vi "Create LVObjectMsg.vi"(8 "error in (no error)":errorcluster, 10 "Message Data":refnum<class>, 11 "Message Name":string) -> (0 "error out":errorcluster, 3 "LVObjectMsg out":refnum<class "LVObjectMsg.lvclass">)   [LabVIEW 2018, in "LapDog.Messaging.v3.NativeTypes.lvlib" / "LVObjectMsg.lvclass"]
doc: "Returns a LVObjectMsg object with the given name.\n\nThis method executes regardless of the error in state."
uses:
  LVObjectMsg.lvclass
  T:/git/LapDog.Messaging/src/LapDog.Messaging/Message/Message.lvclass
  LVObjectMsg.lvclass/LVObjectMsg.ctl
  LapDog.Messaging/Message/Message.lvclass
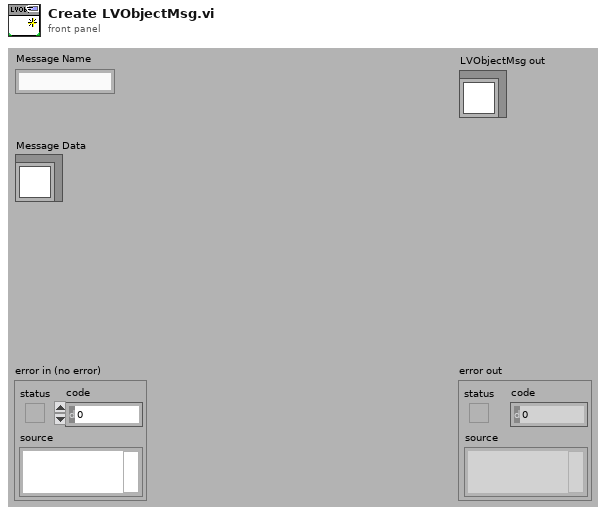
[diagram p1: front panel]
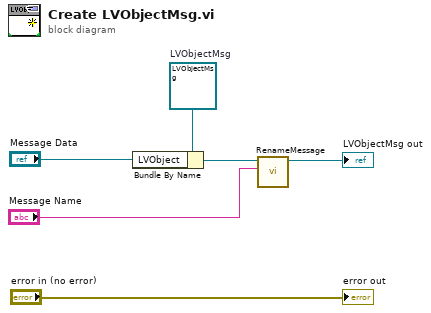
[diagram p0: block diagram]
diagram:
  w1 = refnum<class "LVObjectMsg.lvclass"> refnum  # LVObjectMsg
  n1 = Bundle By Name(cluster=w1, "LVObject"="Message Data") -> (w4:refnum<class "LVObjectMsg.lvclass">)
  n2 = call "RenameMessage.vi"("Message Name"="Message Name", "Message in"=w4) -> ("Message out"=→"LVObjectMsg out":refnum<class "LVObjectMsg.lvclass">)  [unwired: 8 in, 1 out]
  "error out" <- "error in (no error)"
